vi "CRYGet Device Index to Channel.vi"(10 "Device Name In":string, 11 "Device Info In":T1(array[cluster])) -> (1 "Device Total Index Out":i32, 3 "Device Index Out":i32)   [LabVIEW 2013]
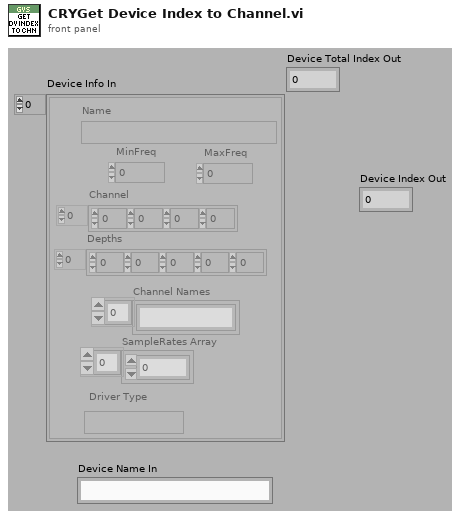
[diagram p1: front panel]
types:
  T1 = cluster{"Name":string, "MinFreq":dbl, "MaxFreq":dbl, "Channel":i32[], "Depths":i32[], "Channel Names":string[], "SampleRates Array":dbl[], "Driver Type":string}[]
  T2 = cluster{"Name":string, "MinFreq":dbl, "MaxFreq":dbl, "Channel":i32[], "Depths":i32[], "Channel Names":string[], "SampleRates Array":dbl[], "Driver Type":string}
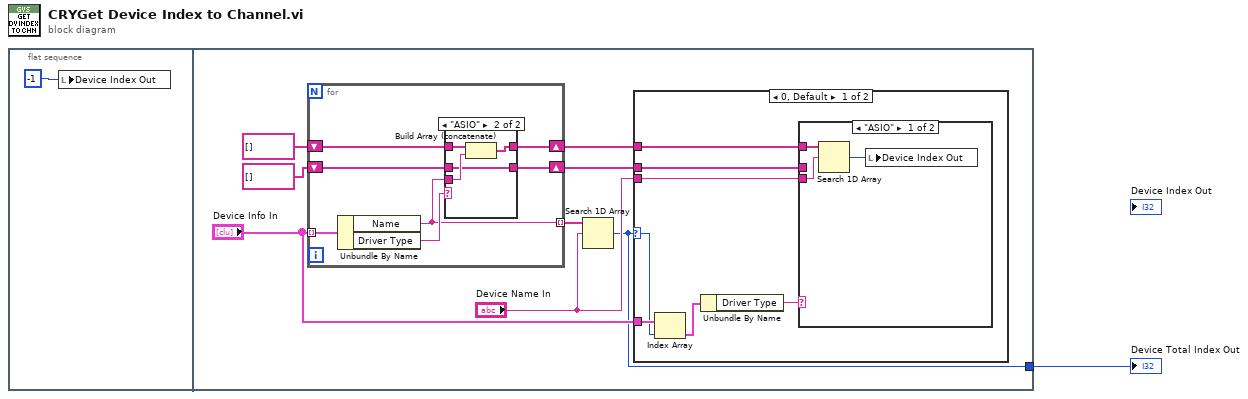
[diagram p0: block diagram]
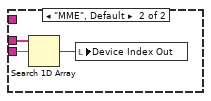
[diagram p2: hidden frame]
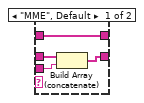
[diagram p4: hidden frame]
diagram:
  n1 = flat-sequence {
    tunnel: [w3] -> w1
    frame #0 {
      n2 = local write "Device Index Out"(-1 ("Device Index Out")) -> ()
    }
    frame #1 {
      n3 = for {
        tunnel: "Device Info In" -> [w30] mode=indexing
        tunnel: [w28] -> w6 mode=indexing
        shift-right: [w25] -> w5
        shift-left: string[] [] -> [w27]
        shift-right: [w24] -> w4
        shift-left: string[] [] -> [w26]
        n4 = Unbundle By Name(w30) -> ("Name"=w28:string, "Driver Type"=w29:string)
        n5 = case shown="\"ASIO\"" w29 {
          tunnel: w28 -> [w33 w38]
          tunnel: w27 -> [w34 w35]
          tunnel: w26 -> [w31 w37]
          tunnel: [w32 w35] -> w25
          tunnel: [w31 w36] -> w24
          frame "MME", Default {
            n6 = Build Array (concatenate)(w34, w33) -> (w32:string[])
          }
          frame "ASIO" {
            n7 = Build Array (concatenate)(w37, w38) -> (w36:string[])
          }
        }
      }
      n8 = Search 1D Array(1D array=w6, element="Device Name In") -> (index of element=w3:i32)  [unwired: 1 in]
      n9 = case shown="0, Default" w3 {
        selector: w3 -> [w16 _]
        tunnel: w5 -> [w13 _]
        tunnel: w4 -> [w12 _]
        tunnel: "Device Name In" -> [w11 _]
        tunnel: "Device Info In" -> [w17 _]
        frame 0, Default {
          n10 = Index Array(array=w17, index=w16) -> (element=w15:T2)
          n11 = Unbundle By Name(w15) -> ("Driver Type"=w14:string)
          n12 = case shown="\"ASIO\"" w14 {
            tunnel: w13 -> [_ w23]
            tunnel: w12 -> [w20 _]
            tunnel: w11 -> [w19 w22]
            frame "ASIO" {
              n13 = Search 1D Array(1D array=w20, element=w19) -> (index of element=w18:i32)  [unwired: 1 in]
              n14 = local write "Device Index Out"(w18) -> ()
            }
            frame "MME", Default {
              n15 = Search 1D Array(1D array=w23, element=w22) -> (index of element=w21:i32)  [unwired: 1 in]
              n16 = local write "Device Index Out"(w21) -> ()
            }
          }
        }
        frame -1 {
        }
      }
    }
  }
  "Device Total Index Out" <- w1
